vi "CAlex2_InitAll.vi"(8 "error in (no error)":errorcluster, 10 "LegProperties":T1={"BodyDim(m)"={"ThighLt"=0.4, "ShankLt"=0.41, "HipWd"=0.32}, "BodyWt(kg)"={"Thigh"=0.0, "Shank"=0.0}, "CuffLoc(m)"={"HipCuffWd"=0.4, "HipCuffHt"=0.1, "HipCuffFwdShift"=0.0, "ThighCuffToKnee"=0.25, "ThighCuffDist"=0.0, "ShankCuffToKnee"=0.15}}, 11 "CAlex2 in":refnum<class "CAlex2.lvclass">) -> (0 "error out":errorcluster, 3 "CAlex2 out":refnum<class "CAlex2.lvclass">)   [LabVIEW 2015, in "CAlex2.lvclass"]
uses:
  CAlex2.lvclass
  TypeDef/LowerBodyDim.ctl
  Body/xyzO.ctl
  <vilib>/Analysis/Matrix/Datatypes/RealMatrix.ctl
  CAlex2.lvclass/CAlex2.ctl
  Body/Bodies.lvclass
  <vilib>/Analysis/Matrix/NI_Matrix.lvlib
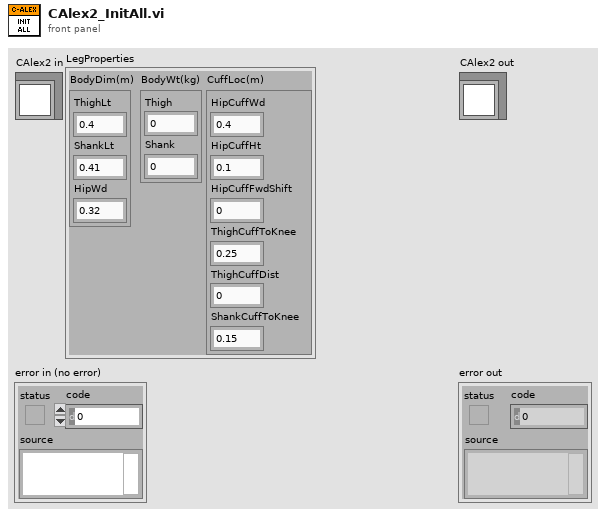
[diagram p1: front panel]
types:
  T1 = typedef "CAlex2.lvclass/LowerBodyDim.ctl" = cluster{"BodyDim(m)":cluster{"ThighLt":dbl, "ShankLt":dbl, "HipWd":dbl}, "BodyWt(kg)":cluster{"Thigh":dbl, "Shank":dbl}, "CuffLoc(m)":cluster{"HipCuffWd":dbl, "HipCuffHt":dbl, "HipCuffFwdShift":dbl, "ThighCuffToKnee":dbl, "ThighCuffDist":dbl, "ShankCuffToKnee":dbl}}
  T2 = typedef "NI_Matrix.lvlib/RealMatrix.ctl" = dbl[][]
  T3 = typedef "Bodies.lvclass/xyzO.ctl" = enum16{"X", "Y", "Z", "O"}
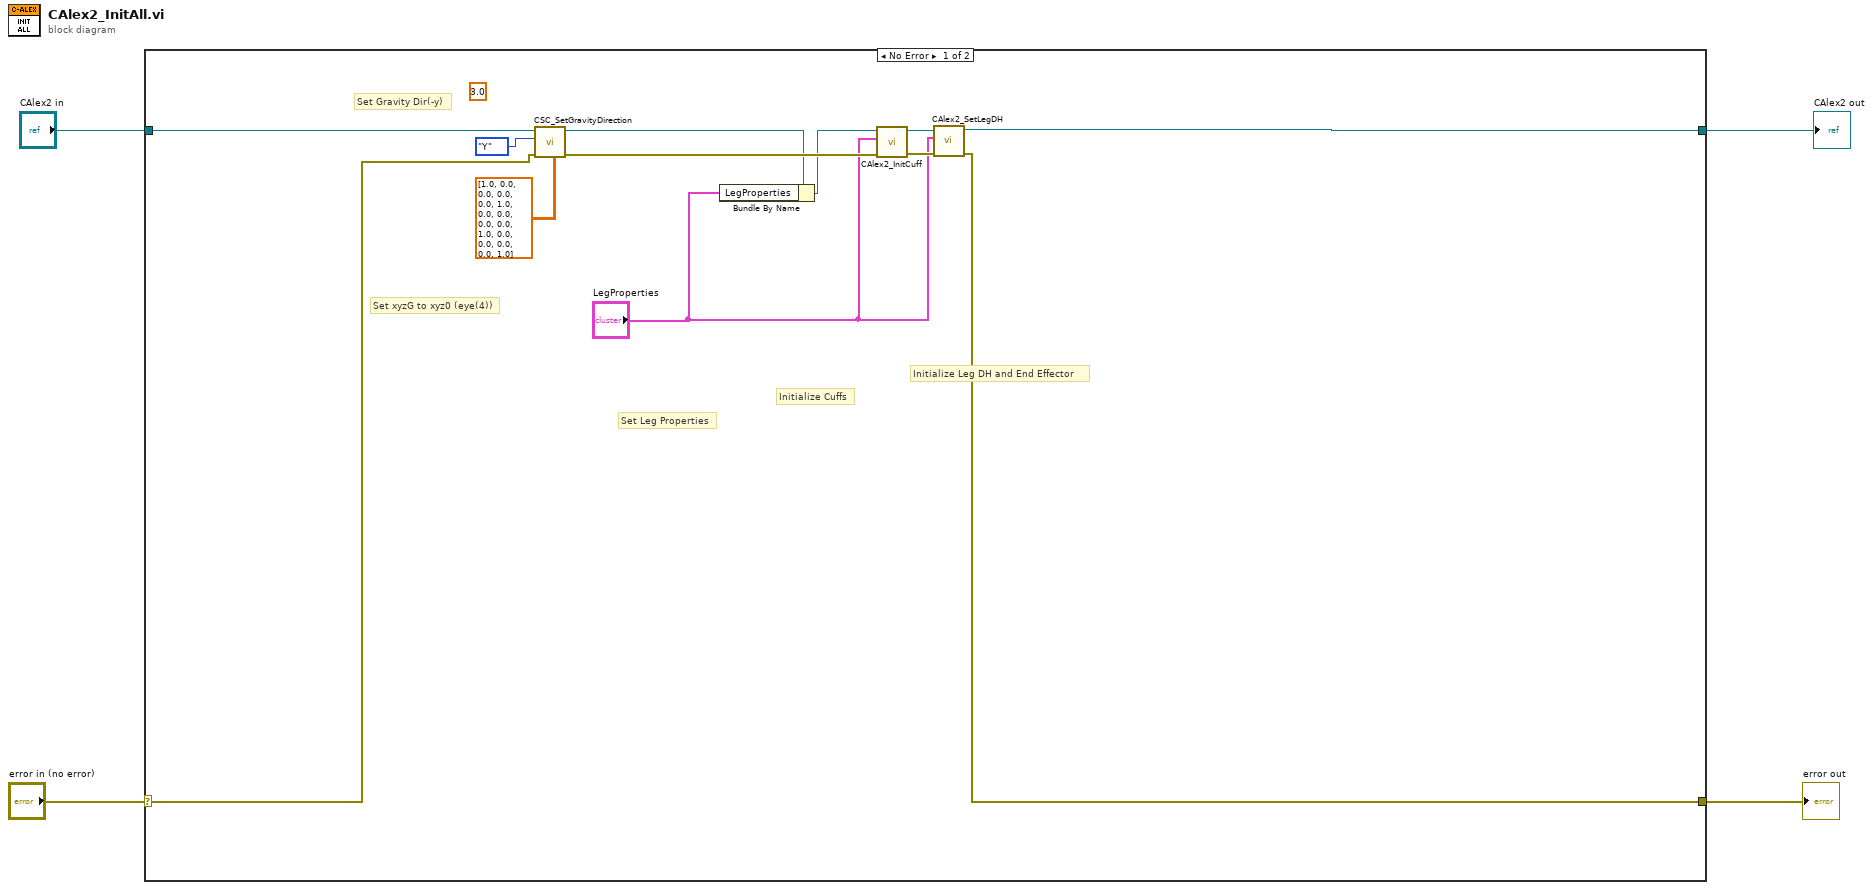
[diagram p0: block diagram]
diagram:
  n1 = case shown="No Error" "error in (no error)" {
    selector: "error in (no error)" -> [w7 w18]
    tunnel: [w6 w18] -> w3
    tunnel: [w13 w17] -> w1
    tunnel: "CAlex2 in" -> [w15 w17]
    frame No Error {
      (unwired) 3.0 ("Numeric")
      # "Initialize Leg DH and End Effector"
      # "Initialize Cuffs"
      # "Set Leg Properties"
      # "Set xyzG to xyz0 (eye(4))"
      # "Set Gravity Dir(-y)"
      n2 = call-dynamic "CSC_SetGravityDirection.vi"("Trans_Gto0"=T2 [[1.0, 0.0, 0.0, 0.0], [0.0, 1.0, 0.0, 0.0], [0.0, 0.0, 1.0, 0.0], [0.0, 0.0, 0.0, 1.0]] ("Trans_0toG"), "error in (no error)"=w7, "Gravity Axis in G (Z)"=xyzO."Y" ("Gravity Axis"), "CSC in"=w15) -> ("error out"=w11:errorcluster, "CSC out"=w10:refnum<class "CAlex2.lvclass">)  [unwired: 6 in]
      n3 = Bundle By Name(cluster=w10, "LegProperties"="LegProperties") -> (w8:refnum<class "CAlex2.lvclass">)
      n4 = call-dynamic "CAlex2_InitCuff.vi"("error in (no error)"=w11, "LegProperty"="LegProperties", "CAlex2 in"=w8) -> ("error out"=w12:errorcluster, "CAlex2 out"=w14:refnum<class "CAlex2.lvclass">)  [unwired: 7 in]
      n5 = call-dynamic "CAlex2_SetLegDH.vi"("error in (no error)"=w12, "ArmProperty"="LegProperties", "CAlex2 in"=w14) -> ("error out"=w6:errorcluster, "CAlex2 out"=w13:refnum<class "CAlex2.lvclass">)  [unwired: 7 in]
    }
    frame Error {
    }
  }
  "error out" <- w3
  "CAlex2 out" <- w1
